vi "set_controls_enabled_state.vi"(8 "error in (no error)":errorcluster, 9 "status":T1(ring), 10 "control references":refnum<vi>[](array[refnum]), 11 "GenericPlugin in":refnum<class "ImagingModeMG090624Camera.lvclass">) -> (0 "error out":errorcluster, 3 "GenericPlugin out":refnum<class "ImagingModeMG090624Camera.lvclass">)   [LabVIEW 2010, in "ImagingModeMG090624Camera.lvclass"]
uses:
  ImagingModeMG090624Camera.lvclass
  ImagingModeDL091001Scaffold/ImagingModeDL091001Scaffold/ImagingModeDL091001Scaffold.lvclass
  ImagingModeMG090624Camera.lvclass/ImagingModeMG090624Camera.ctl
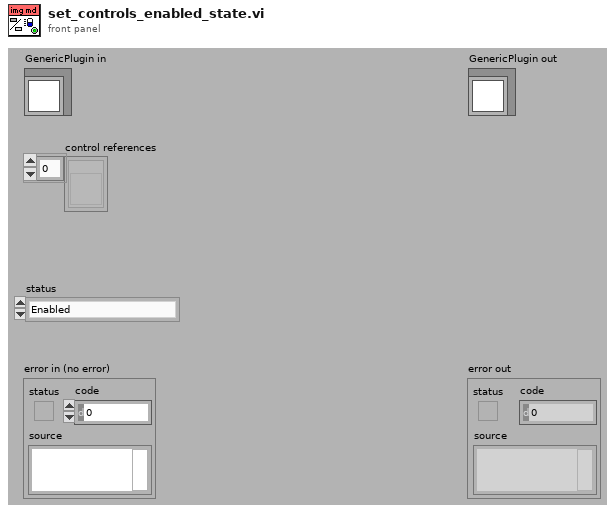
[diagram p1: front panel]
types:
  T1 = enum8{"Enabled", "Disabled", "Disabled and Grayed Out"}
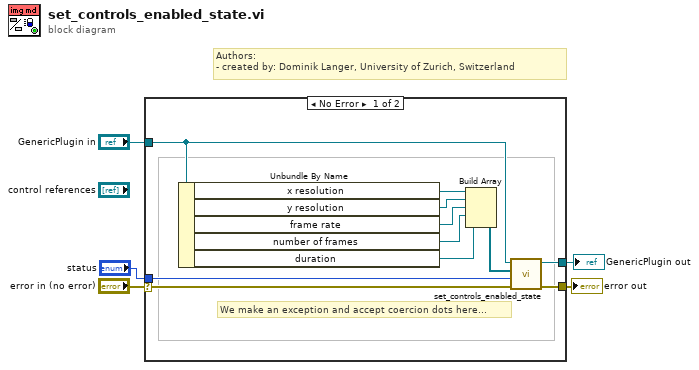
[diagram p0: block diagram]
diagram:
  # "Authors: \n- created by: Dominik Langer, University of Zurich, Switzerland"
  n1 = case shown="No Error" "error in (no error)" {
    selector: "error in (no error)" -> [w6 w17]
    tunnel: [w16 w17] -> w5
    tunnel: [w15 w18] -> w4
    tunnel: "status" -> [w14 _]
    tunnel: "GenericPlugin in" -> [w13 w18]
    frame No Error {
      # "We make an exception and accept coercion dots here..."
      n2 = Unbundle By Name(w13) -> ("x resolution"=w12:refnum<vi>, "y resolution"=w11:refnum<vi>, "frame rate"=w10:refnum<vi>, "number of frames"=w9:refnum<vi>, "duration"=w8:refnum<vi>)
      n3 = Build Array(w12, w11, w10, w9, w8) -> (w7:refnum<vi>[])
      n4 = call-parent "set_controls_enabled_state.vi"("error in (no error)"=w6, "status"=w14, "control references"=w7, "GenericPlugin in"=w13) -> ("error out"=w16:errorcluster, "GenericPlugin out"=w15:refnum<class "ImagingModeMG090624Camera.lvclass">)  [unwired: 6 in]
    }
    frame Error {
    }
  }
  "error out" <- w5
  "GenericPlugin out" <- w4
